vi "Initialize.vi"(8 "error in (no error)":errorcluster, 9 "Requestor":string, 10 "Requestee":string, 11 "Mag Lab Root in":refnum<class "Mag Lab Root.lvclass">) -> (0 "error out":errorcluster, 3 "Mag Lab Root out":refnum<class "Mag Lab Root.lvclass">)   [LabVIEW 2015, in "Mag Lab Root.lvclass"]
uses:
  Mag Lab Root.lvclass
  Mag Lab Root.lvclass/Mag Lab Root.ctl
  <vilib>/ActorFramework/Actor/Actor.lvclass/Actor.ctl
  Mag Lab Root Messages/Recieve Acknowledge Initialized Msg/Recieve Acknowledge Initialized Msg.lvclass/Recieve Acknowledge Initialized Msg.ctl
  <vilib>/ActorFramework/Message Enqueuer/Message Enqueuer.lvclass/Message Enqueuer.ctl
  <vilib>/ActorFramework/Message Enqueuer/Enqueue.vi
  <vilib>/ActorFramework/Message Priority Queue/Priority Enqueue.vi
  Mag Lab Root Messages/Recieve Acknowledge Initialized Msg/Recieve Acknowledge Initialized Msg.lvclass
  <vilib>/ActorFramework/Actor/Actor.lvclass
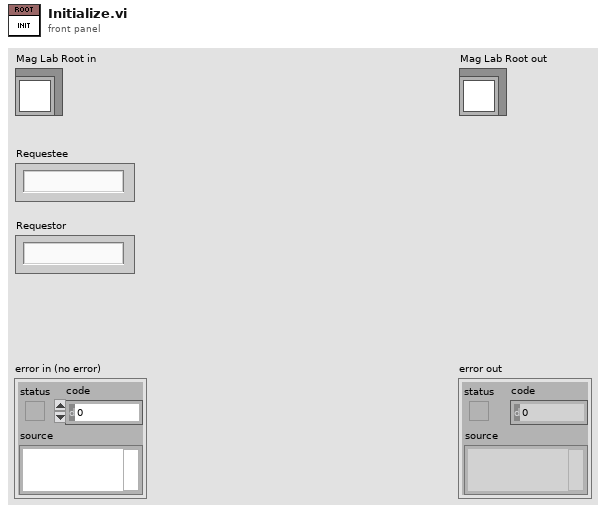
[diagram p1: front panel]
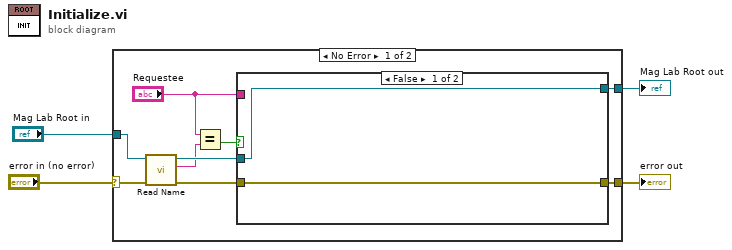
[diagram p0: block diagram]
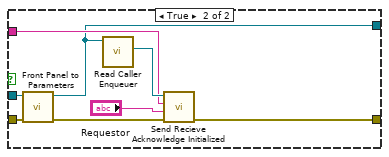
[diagram p2: hidden frame]
diagram:
  n1 = case shown="No Error" "error in (no error)" {
    selector: "error in (no error)" -> [w8 w25]
    tunnel: [w13 w25] -> w3
    tunnel: [w7 w24] -> w1
    tunnel: "Mag Lab Root in" -> [w6 w24]
    frame No Error {
      n2 = call "Read Name.vi"("error in (no error)"=w8, "Mag Lab Root in"=w6) -> ("error out"=w11:errorcluster, "Name"=w10:string, "Mag Lab Root out"=w12:refnum<class "Mag Lab Root.lvclass">)  [unwired: 7 in]
      n3 = Equal?(x="Requestee", y=w10) -> (x = y?=w5:bool)
      n4 = case shown="False" w5 {
        tunnel: [w14 w22] -> w13
        tunnel: w12 -> [w15 w20]
        tunnel: w11 -> [w14 w19]
        tunnel: "Requestee" -> [_ w18]
        tunnel: [w15 w16] -> w7
        frame False {
        }
        frame True {
          n5 = call-dynamic "Front Panel to Parameters.vi"("error in (no error)"=w19, "Mag Lab Root in"=w20) -> ("error out"=w17:errorcluster, "Mag Lab Root out"=w16:refnum<class "Mag Lab Root.lvclass">)  [unwired: 8 in]
          n6 = call <vilib>:"Read Caller Enqueuer.vi"("Actor"=w16) -> ("Caller Enqueuer"=w21:refnum<class "Message Enqueuer.lvclass">)  [unwired: 10 in]
          n7 = call "Send Recieve Acknowledge Initialized.vi"("error in (no error)"=w17, "Requestor"="Requestor", "Requestee"=w18, "Message Enqueuer"=w21) -> ("error out"=w22:errorcluster)  [unwired: 6 in, 1 out]
        }
      }
    }
    frame Error {
    }
  }
  "error out" <- w3
  "Mag Lab Root out" <- w1
